vi "L1_fifttyIPRFinder.vi"(0 "VISA In":refnum<visa-resource-name>="AgilentOsciloscope", 1 "Channel Register":i32=97, 2 "Vin":dbl=0.4, 3 "File path In":path=path "C:/Users/omartinez/Desktop/L0nL1_Results/L1_SN_test_DT_Test.csv", 5 "ID In":refnum<k5>, 7 "Error In":errorcluster, 9 "Array":i16[](array[numeric])=[0, 200], 11 "CH":i32=3, 12 "Active Adder":i32=97, 13 "IPR Register Read Select":i32) -> (4 "VISA Out":refnum<visa-resource-name>="AgilentOsciloscope", 6 "ID out":refnum<k5>, 8 "Error Out":errorcluster={"status"=TRUE, "code"=1, "source"="TCP Write in send_receive(SubVI).vi->sendCommand.vi->spi_full_control.vi->Single_ASIC_L1_R_W.vi->L1_fifttyIPRFinder.vi"}, 10 "Array 2":i16[](array[numeric])=[0, 1])   [LabVIEW 2012]
uses:
  Sum_Abrilader/L0_Sum_Adder Folder/C/Program Files/National Instruments/LabVIEW 2012/instr.lib/Agilent 8000 Series/Public/Data/Low Level/Fetch Measurement (More).vi
  <instrlib>/Agilent 8000 Series/Agilent 8000 Series.lvlib
panel:
  out "IPR_count":u32
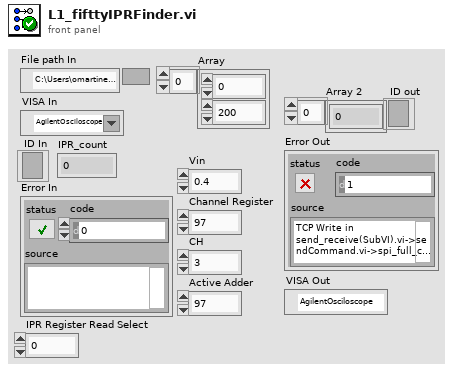
[diagram p1: front panel]
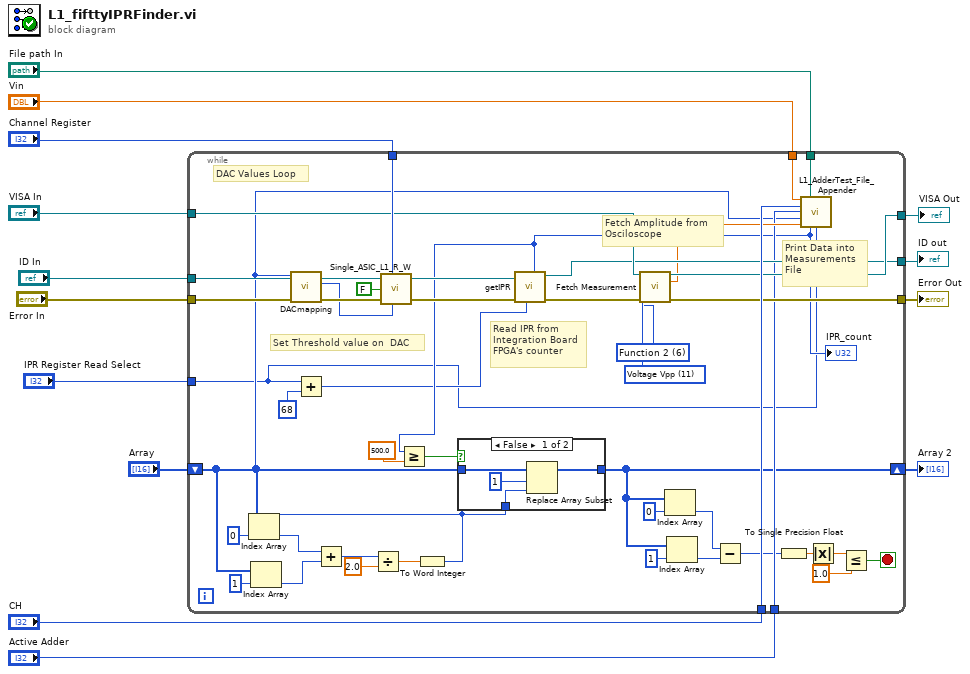
[diagram p0: block diagram]
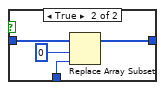
[diagram p2: hidden frame]
diagram:
  n1 = while {
    tunnel: "ID In" -> [w59]
    tunnel: "Channel Register" -> [w57]
    tunnel: "Error In" -> [w56]
    tunnel: [w42] -> w8
    tunnel: [w48] -> w9
    tunnel: "File path In" -> [w53]
    tunnel: "CH" -> [w52]
    tunnel: "Active Adder" -> [w40]
    tunnel: "Vin" -> [w51]
    tunnel: "VISA In" -> [w47]
    tunnel: [w46] -> w7
    shift-right: [w20] -> w10
    shift-left: "Array" -> [w25]
    tunnel: "IPR Register Read Select" -> [w15]
    stop <- w24 stop-if-true
    w50 = 11 items=["Rise Time", "Fall Time", "Frequency", "Period", "Voltage RMS(AC)", "Voltage RMS(DC)", "Voltage RMS (AC,cycle)", "Voltage RMS (DC,cycle)", "Voltage Max", "Voltage Min", "Voltage Middle", "Voltage Vpp", "Voltage High", "Voltage Low", "Voltage Average", "Voltage Average (cycle)", "Width Negative", "Width Positive", "Duty Cycle Positive", "Amplitude", "Overshoot", "Preshoot", "Voltage Base", "Voltage Upper", "Time Max", "Time Min", "Color Grade Crossing", "Color Grade Eye Width", "Color Grade Eye Height", "Color Grade Eye Q-Factory", "Color Grade Eye Duty Cycle Distortion(Percent)", "Color Grade Eye Duty Cycle Distortion(Time)", "Color Grade Eye Jitter(PP)", "Color Grade Eye Width(RMS)", "Cycle-cycle Duty Jitter(Rising)", "Cycle-cycle Duty Jitter(Falling)", "Cycle-cycle Jitter(Rising)", "Cycle-cycle Jitter(Falling)", "Cycle-cycle - Width", "Cycle-cycle + Width", "Date Rate", "Unit Interval", "FFT Delta Frequency", "FFT Delta Magnitude", "FFT Frequency", "FFT Magnitude", "Slew Rate", "Area (Entire Display)", "Area(Single Cycle)", "Duty Cycle (Rising)", "Duty Cycle (Falling)"] ("Measurement Function (0: Rise Time)")
    w49 = 6 items=["Channel 1"=1, "Channel 2"=2, "Channel 3"=3, "Channel 4"=4, "Function 1"=5, "Function 2"=6, "Function 3"=7, "Function 4"=8, "Memory 1"=9, "Memory 2"=10, "Memory 3"=11, "Memory 4"=12] ("Channel (1: Channel 1)")
    # "Print Data into\nMeasurements \nFile"
    # "Fetch Amplitude from\nOsciloscope"
    # "Read IPR from \nIntegration Board\nFPGA's counter"
    # "Set Threshold value on  DAC"
    # "DAC Values Loop"
    n2 = Index Array(array=w25, index=0) -> (element=w32:i16)
    n3 = Index Array(array=w25, index=1) -> (element=w31:i16)
    n4 = Add(x=w15, y=68) -> (x+y=w17:i32)
    n5 = Add(x=w32, y=w31) -> (x+y=w37:i16)
    n6 = Divide(x=w37, y=2.0) -> (x/y=w33:dbl)
    n7 = To Word Integer(number=w33) -> (16bit integer=w23:i16)
    n8 = call "DACmapping.vi"("error in (no error)"=w56, "DAC_TH"=w23) -> ("error out"=w55:errorcluster, "COMB DEC"=w54:u32)  [unwired: 8 in]
    n9 = call "Single_ASIC_L1_R_W.vi"("connection ID"=w59, "Register or channel"=w57, "RD/#WR"=FALSE, "error in (no error)"=w55, "Data"=w54) -> ("connection ID out"=w43:refnum<k5>, "error out"=w45:errorcluster)  [unwired: 1 in, 2 out]
    n10 = call "getIPR.vi"("Address"=w17, "error in"=w45, "connection ID"=w43) -> ("error out"=w44:errorcluster, "connection ID out"=w42:refnum<k5>, "IPR_count"=w26:u32)  [unwired: 5 in, 1 out]
    "IPR_count" <- w26
    n11 = Greater Or Equal?(x=w26, y=500.0) -> (x >= y?=w34:bool)
    n12 = case shown="False" w34 {
      tunnel: w25 -> [w61 w66]
      tunnel: [w60 w67] -> w20
      tunnel: w23 -> [w63 w64]
      frame False {
        n13 = Replace Array Subset(array=w61, new element=w63, index=1) -> (w60:i16[])
      }
      frame True {
        n14 = Replace Array Subset(array=w66, new element=w64, index=0) -> (w67:i16[])
      }
    }
    n15 = call-poly "Fetch Measurement.vi"("VISA resource name"=w47, "Channel (1: Channel 1)"=w49, "Measurement Function (0: Rise Time)"=w50, "error in (no error)"=w44) -> ("VISA resource name out"=w46:refnum<visa-resource-name>, "Measurement"=w41:dbl, "error out"=w48:errorcluster)  [unwired: 9 in]
    n16 = Index Array(array=w20, index=0) -> (element=w19:i16)
    n17 = Index Array(array=w20, index=1) -> (element=w18:i16)
    n18 = Subtract(x=w19, y=w18) -> (x-y=w30:i16)
    n19 = To Single Precision Float(number=w30) -> (single precision float=w29:sgl)
    n20 = call "L1_AdderTest_File_Appender.vi"("Vin"=w51, "file path (dialog if empty)"=w53, "CH"=w52, "Active Adder"=w40, "DAC Level"=w23, "Vmeas"=w41, "IPR"=w26, "Digital Output"=w15) -> ()  [unwired: 8 in]
    n21 = Absolute Value(x=w29) -> (abs(x)=w28:sgl)
    n22 = Less Or Equal?(x=w28, y=sgl 1.0) -> (x <= y?=w24:bool)
  }
  "Array 2" <- w10
  "Error Out" <- w9
  "ID out" <- w8
  "VISA Out" <- w7
